vi "Allocate.vi"(8 "Error In":errorcluster, 11 "Capacity":u32) -> (0 "Error Out":errorcluster, 3 "ByteBuffer Out":refnum<class "ByteBuffer.lvclass">)   [LabVIEW 2015, in "ByteBuffer.lvclass"]
doc: "Allocates a new direct byte buffer.\nThe new buffer's position will be zero, its limit will be its capacity, its mark will be undefined, and each of its elements will be initialized to zero. Whether or not it has a backing array is unspecified.\n\nParameters:\n+ Capacity - The new buffer's capacity, in bytes.\n\nReturns:\nThe new byte buffer.\n\nThrows:\n+ IllegalArgumentException - If the capacity is a negative integer."
uses:
  ByteBuffer.lvclass
  ByteBuffer.lvclass/ByteBuffer.ctl
  <vilib>/Utility/error.llb/Error Cluster From Error Code.vi
  <vilib>/ErrorRing/Error Ring.xnode
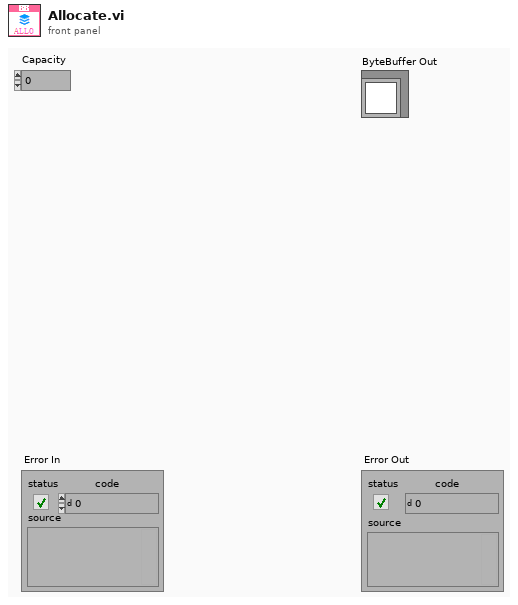
[diagram p1: front panel]
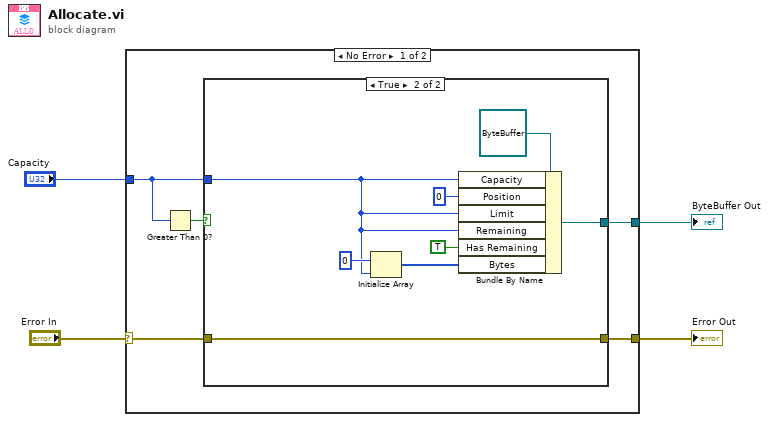
[diagram p0: block diagram]
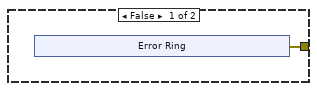
[diagram p2: hidden frame]
diagram:
  n1 = case shown="No Error" "Error In" {
    selector: "Error In" -> [w6 w24]
    tunnel: "Capacity" -> [w7 _]
    tunnel: [w5 w24] -> w2
    tunnel: [w9 _] -> w1
    frame No Error {
      n2 = Greater Than 0?(x=w7) -> (x > 0?=w8:bool)
      n3 = case shown="True" w8 {
        tunnel: w7 -> [_ w16]
        tunnel: [_ w18] -> w9
        tunnel: w6 -> [_ w17]
        tunnel: [w10 w17] -> w5
        frame False {
          n4 = xnode "Error Ring"() -> ("error out"=w10:errorcluster)
        }
        frame True {
          n5 = Initialize Array(u8 0, w16) -> (w19:u8[])
          n6 = Bundle By Name(cluster=refnum<class "ByteBuffer.lvclass"> refnum ("ByteBuffer Out"), "Capacity"=w16, "Position"=u32 0, "Limit"=w16, "Remaining"=w16, "Has Remaining"=TRUE, "Bytes"=w19) -> (w18:refnum<class "ByteBuffer.lvclass">)
        }
      }
    }
    frame Error {
    }
  }
  "ByteBuffer Out" <- w1
  "Error Out" <- w2
